vi "OP500ZP_ADJ.vi"(8 "errin":errorcluster caption="entrée d'erreur (pas d'erreur)", 10 "BT3562A":string(combo) caption="Nom de ressource VISA") -> (0 "errout":errorcluster caption="sortie d'erreur", 2 "ADJ?":bool)   [LabVIEW 2020]
uses:
  16daea3c-e4e3-4f5e-a176-e24f6f152e7e.vi
  ff3bc6fb-eb8a-4911-8f19-68f4c64bebaa.vi
  <vilib>/Instr/_visa.llb/VISA Configure Serial Port (Instr).vi
  <instrlib>/HIOKI BT356X Series/HIOKI BT356X Series.lvlib
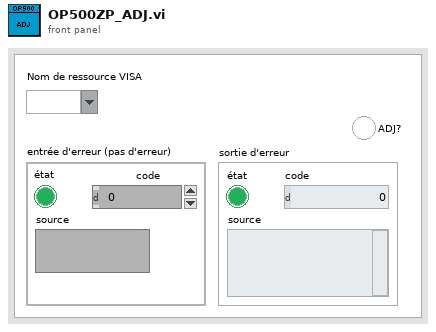
[diagram p1: front panel]
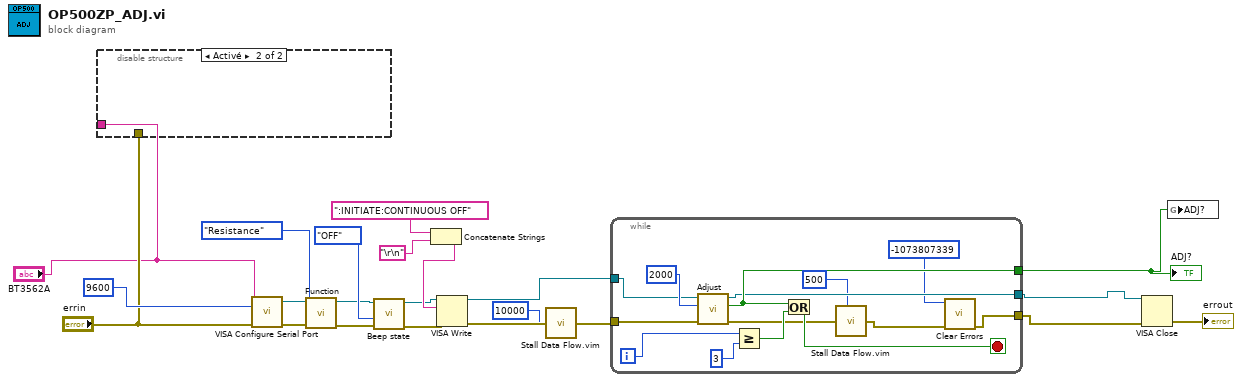
[diagram p0: block diagram]
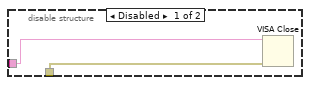
[diagram p2: hidden frame]
diagram:
  n1 = disable-structure shown="Activé" {
    disable-tunnel: "BT3562A" -> [w24 _]
    disable-tunnel: "errin" -> [w23 _]
    frame Disabled {
      n2 = VISA Close(VISA resource name=w24, error in (no error)=w23) -> ()  [unwired: 1 out]
    }
    frame Enabled {
    }
  }
  n3 = call-poly "VISA Configure Serial Port"("VISA resource name"="BT3562A", "baud rate (9600)"=u32 9600, "error in (no error)"="errin") -> ("VISA resource name out"=w15:refnum<visa-resource-name>, "error out"=w16:errorcluster)  [unwired: 11 in]
  n4 = call <instrlib>:"Function.vi"("error in (no error)"=w16, "Function set"=enum16{"RV", "Resistance", "Voltage"}."Resistance", "VISA session"=w15) -> ("error out"=w10:errorcluster, "dup VISA session"=w12:refnum<visa-resource-name>)  [unwired: 6 in, 1 out]
  n5 = call <instrlib>:"Beep state.vi"("error in (no error)"=w10, "Beep set"=enum16{"ON", "OFF"}."OFF", "VISA session"=w12) -> ("error out"=w9:errorcluster, "dup VISA session"=w11:refnum<visa-resource-name>)  [unwired: 6 in, 1 out]
  n6 = Concatenate Strings(":INITIATE:CONTINUOUS OFF" ("buffer d'écriture"), "\r\n") -> (w19:string)
  n7 = VISA Write(VISA resource name=w11, write buffer=w19, error in (no error)=w9) -> (VISA resource name out=w3:refnum<visa-resource-name>, error out=w4:errorcluster)  [unwired: 1 out]
  n8 = call "Stall Data Flow.vim"("value in"=w4, "milliseconds to wait"=u32 10000) -> ("value out"=w5:errorcluster)  [unwired: 1 out]
  n9 = while {
    tunnel: [w37] -> w8
    tunnel: [w26] -> w6
    tunnel: [w34] -> w7
    tunnel: w5 -> [w33]
    tunnel: w3 -> [w25]
    i -> [w30]
    stop <- w35 stop-if-true
    n10 = call <instrlib>:"Adjust.vi"("error in (no error)"=w33, "Timeout Value"=u32 2000, "VISA session"=w25) -> ("error out"=w32:errorcluster, "Complete"=w37:bool, "dup VISA session"=w34:refnum<visa-resource-name>)  [unwired: 6 in]
    n11 = Greater Or Equal?(x=w30, y=3 ("x")) -> (x >= y?=w36:bool)
    n12 = Or(x=w37, y=w36) -> (x .or. y?=w35:bool)
    n13 = call "Stall Data Flow.vim"("value in"=w32, "milliseconds to wait"=u32 500) -> ("value out"=w27:errorcluster)  [unwired: 1 out]
    n14 = call <vilib>:"Clear Errors.vi"("error in (no error)"=w27, "specific error code to clear (0: all)"=-1073807339) -> ("error out"=w26:errorcluster)  [unwired: 4 in, 1 out]
  }
  "ADJ?" <- w8
  n15 = VISA Close(VISA resource name=w7, error in (no error)=w6) -> (error out=→"errout":errorcluster)
  n16 = global write "ADJ" "ADJ?"(w8) -> ()
